vi "GDSString_EvaluateMethodText.vi"(0 "MethodString":string) -> (14 "MethodName":string, 15 "FirstArgumentString(Input)":string, 16 "SecondArgumentString(Output)":string, 17 "Scope/Visibility":T1, 18 "Likely a Modifing Methods":bool, 19 "MethodAttributeName":string)   [LabVIEW 2020]
uses:
  <resource>/Framework/Providers/Open_GDS/ClassProviders/Provider_EndevoGOOP300/GOOP300_SubVIs/GOOP300_MethodScopeType.ctl
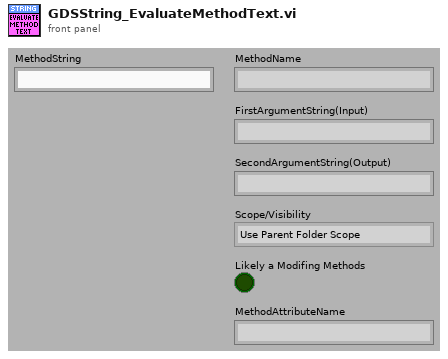
[diagram p1: front panel]
types:
  T1 = typedef "GOOP300_MethodScopeType.ctl" = enum16{"Use Parent Folder Scope", "Public", "Protected", "Private", "Community"}
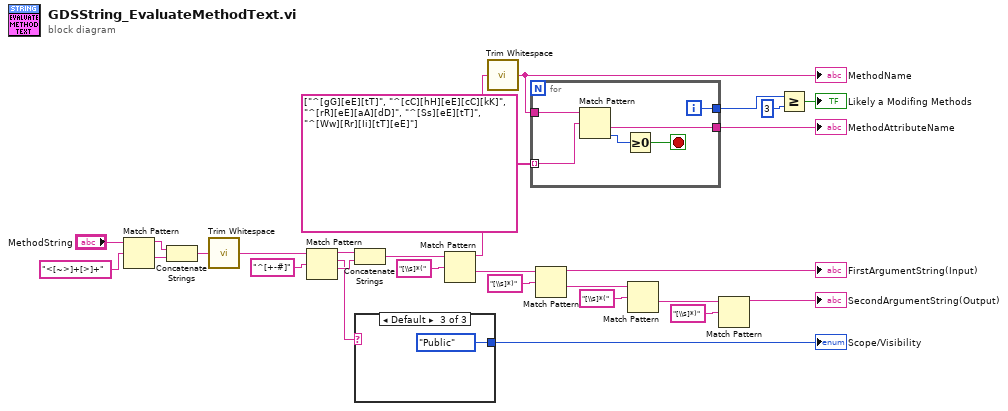
[diagram p0: block diagram]
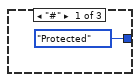
[diagram p2: hidden frame]
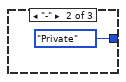
[diagram p3: hidden frame]
diagram:
  n1 = Match Pattern(string="MethodString", regular expression="<[~>]+[>]+") -> (before substring=w16:string, after substring=w17:string)  [unwired: 3 out]
  n2 = Concatenate Strings(w16, w17) -> (w15:string)
  n3 = call <vilib>:"Trim Whitespace.vi"("string"=w15) -> ("trimmed string"=w26:string)  [unwired: 1 in]
  n4 = Match Pattern(string=w26, regular expression="^[+-#]") -> (before substring=w21:string, match substring=w11:string, after substring=w22:string)  [unwired: 2 out]
  n5 = Concatenate Strings(w21, w22) -> (w24:string)
  n6 = case shown="Default" w11 {
    tunnel: [GOOP300_MethodScopeType."Protected" ("Scope/Visibility") GOOP300_MethodScopeType."Private" ("Scope/Visibility") GOOP300_MethodScopeType."Public" ("Scope/Visibility")] -> w10
    frame "#" {
    }
    frame "-" {
    }
    frame Default {
    }
  }
  "Scope/Visibility" <- w10
  n7 = Match Pattern(string=w24, regular expression="[\\s]*(") -> (before substring=w27:string, after substring=w9:string)  [unwired: 3 out]
  n8 = call <vilib>:"Trim Whitespace.vi"("string"=w27) -> ("trimmed string"=w28:string)  [unwired: 1 in]
  "MethodName" <- w28
  n9 = for {
    tunnel: w28 -> [w36]
    tunnel: string[] ["^[gG][eE][tT]", "^[cC][hH][eE][cC][kK]", "^[rR][eE][aA][dD]", "^[Ss][eE][tT]", "^[Ww][Rr][Ii][tT][eE]"] -> [w35] mode=indexing
    tunnel: [w33] -> w14
    tunnel: [w32] -> w12
    i -> [w33]
    stop <- w34 stop-if-true
    n10 = Match Pattern(string=w36, regular expression=w35) -> (after substring=w32:string, offset past match=w37:i32)  [unwired: 3 out]
    n11 = Greater Or Equal To 0?(x=w37) -> (x >= 0?=w34:bool)
  }
  "MethodAttributeName" <- w12
  n12 = Match Pattern(string=w9, regular expression="[\\s]*)") -> (before substring=→"FirstArgumentString(Input)":string, after substring=w5:string)  [unwired: 3 out]
  n13 = Match Pattern(string=w5, regular expression="[\\s]*(") -> (after substring=w2:string)  [unwired: 4 out]
  n14 = Match Pattern(string=w2, regular expression="[\\s]*)") -> (before substring=→"SecondArgumentString(Output)":string)  [unwired: 4 out]
  n15 = Greater Or Equal?(x=w14, y=3) -> (x >= y?=→"Likely a Modifing Methods":bool)
